vi "beta.vi"(2 "alpha":dbl=10.0 format="%#_16g", 3 "NuOptRe":dbl format="%#_16g", 4 "GammaD":dbl format="%#_16g") -> (0 "nuR":dbl format="%#_16g", 1 "beta":dbl format="%#_16g")   [LabVIEW 2015]
panel:
  # "Beta-Correction Function"
  # "Subroutine to compute beta-correction used for hard-collision based line-shape profiles to correct NuOptRe value in the profile. Applicable up to alpha = 5.0, for higher alpha values correction neglected. \nSource: 10.1016/j.jqsrt.2019.106784\n\nStandard Input Parameters:\n--------------------\nGammaD  : Doppler broadening in cm-1. \nNuOptRe : Real part of the Dicke parameter in cm-1.\nalpha   : Mass ratio in the molecule, applicable up to alpha=5, dimensionless.\n\nThe function has one output:\n--------------------\n(1)       : Value of the beta correction, dimensionless."
  # "Output Section"
  # "Input Section"
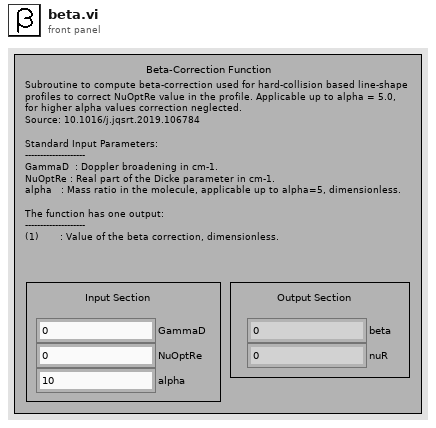
[diagram p1: front panel]
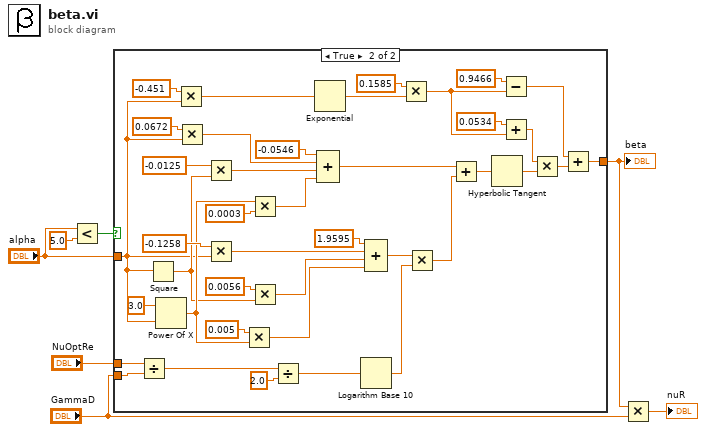
[diagram p0: block diagram]
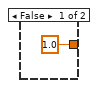
[diagram p2: hidden frame]
diagram:
  n1 = Less?(x="alpha", y=5.0) -> (x < y?=w2:bool)
  n2 = case shown="True" w2 {
    tunnel: [1.0 w12] -> w7
    tunnel: "alpha" -> [_ w11]
    tunnel: "NuOptRe" -> [_ w10]
    tunnel: "GammaD" -> [_ w9]
    frame False {
    }
    frame True {
      n3 = Divide(x=w10, y=w9) -> (x/y=w24:dbl)
      n4 = Square(x=w11) -> (x^2=w34:dbl)
      n5 = Power Of X(1:w11, 2:3.0 ("y")) -> (0:w36:dbl)
      n6 = Multiply(x=-0.451, y=w11) -> (x*y=w46:dbl)
      n7 = Multiply(x=0.0672, y=w11) -> (x*y=w27:dbl)
      n8 = Multiply(x=-0.0125, y=w34) -> (x*y=w26:dbl)
      n9 = Multiply(x=-0.1258, y=w11) -> (x*y=w31:dbl)
      n10 = Multiply(x=0.005, y=w36) -> (x*y=w29:dbl)
      n11 = Multiply(x=w36, y=0.0003) -> (x*y=w25:dbl)
      n12 = Multiply(x=0.0056, y=w34) -> (x*y=w30:dbl)
      n13 = Divide(x=w24, y=2.0) -> (x/y=w22:dbl)
      n14 = Exponential(1:w46) -> (0:w45:dbl)
      n15 = Compound Arithmetic op=ADD(-0.0546, w27, w26, w25) -> (w18:dbl)
      n16 = Logarithm Base 10(1:w22) -> (0:w20:dbl)
      n17 = Compound Arithmetic op=ADD(1.9595, w31, w30, w29) -> (w21:dbl)
      n18 = Multiply(x=0.1585, y=w45) -> (x*y=w42:dbl)
      n19 = Multiply(x=w21, y=w20) -> (x*y=w19:dbl)
      n20 = Add(x=w18, y=w19) -> (x+y=w17:dbl)
      n21 = Hyperbolic Tangent(1:w17) -> (0:w16:dbl)
      n22 = Subtract(x=0.9466, y=w42) -> (x-y=w13:dbl)
      n23 = Add(x=0.0534, y=w42) -> (x+y=w15:dbl)
      n24 = Multiply(x=w15, y=w16) -> (x*y=w14:dbl)
      n25 = Add(x=w13, y=w14) -> (x+y=w12:dbl)
    }
  }
  "beta" <- w7
  n26 = Multiply(x=w7, y="GammaD") -> (x*y=→"nuR":dbl)
